vi "API_BINANCE_Execute_Function.vi"(0 "BinanceAPI in":refnum<class "BinanceAPI_.lvclass">, 11 "error in (no error)":errorcluster) -> (4 "BinanceAPI out":refnum<class "BinanceAPI_.lvclass">, 6 "Header":string, 8 "Body":string, 14 "REST API URL":string, 15 "error out":errorcluster)   [LabVIEW 2022 SP3, in "BinanceAPI_.lvclass"]
uses:
  BinanceAPI_.lvclass
  BinanceAPI_.lvclass/BinanceAPI_.ctl
  <vilib>/httpClient/PUTBuffer.vi
  <vilib>/httpClient/POSTBuffer.vi
  <vilib>/University of Leeds/SHA256/SHA256.lvlib
  <vilib>/httpClient/LabVIEWHTTPClient.lvlib
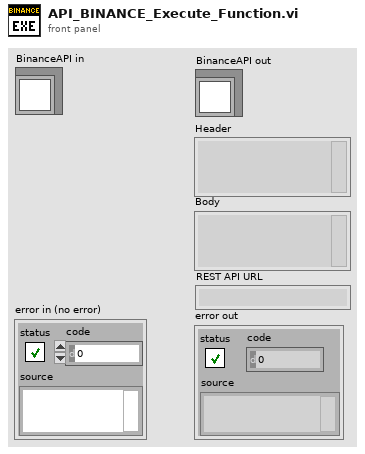
[diagram p1: front panel]
types:
  T1 = enum16{"SPOT", "USDT_FUTURES", "COIN_FUTURES", "VANILLA"}
  T2 = typedef "LabVIEWHTTPClient.lvlib/ClientHandle.ctl" = refnum<k1>
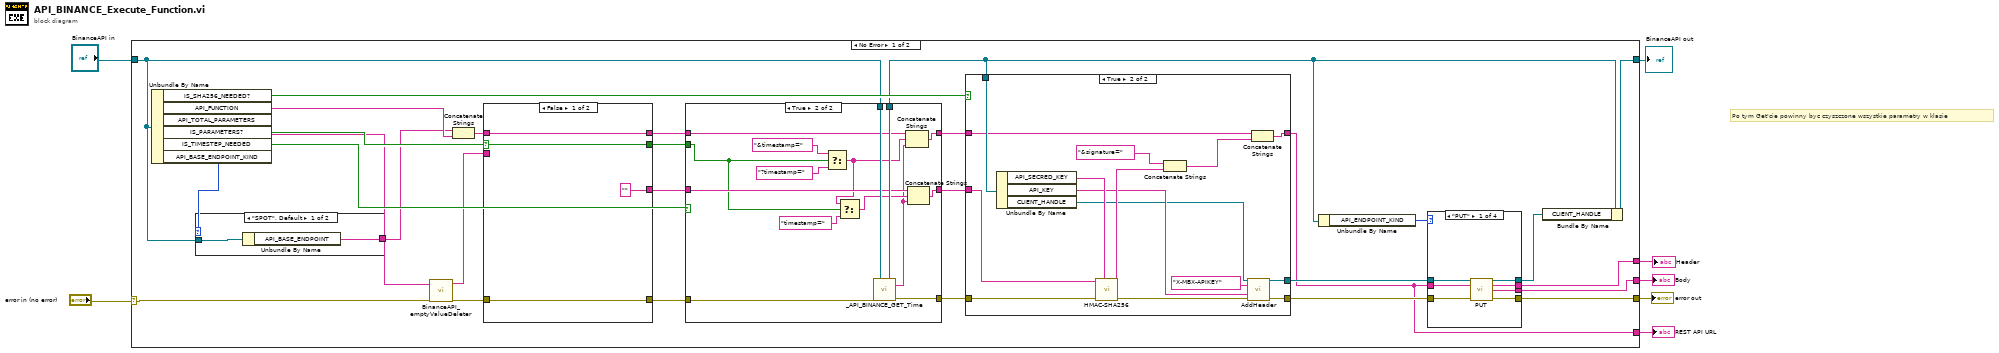
[diagram p0: block diagram]
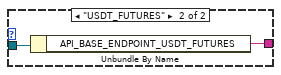
[diagram p2: hidden frame]
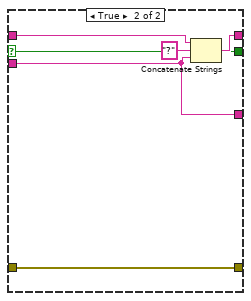
[diagram p4: hidden frame]
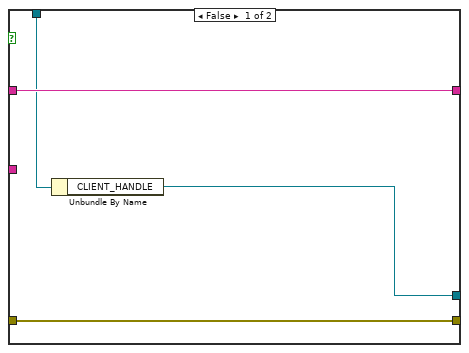
[diagram p5: hidden frame]
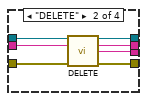
[diagram p6: hidden frame]
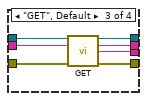
[diagram p7: hidden frame]
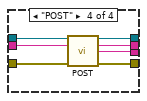
[diagram p8: hidden frame]
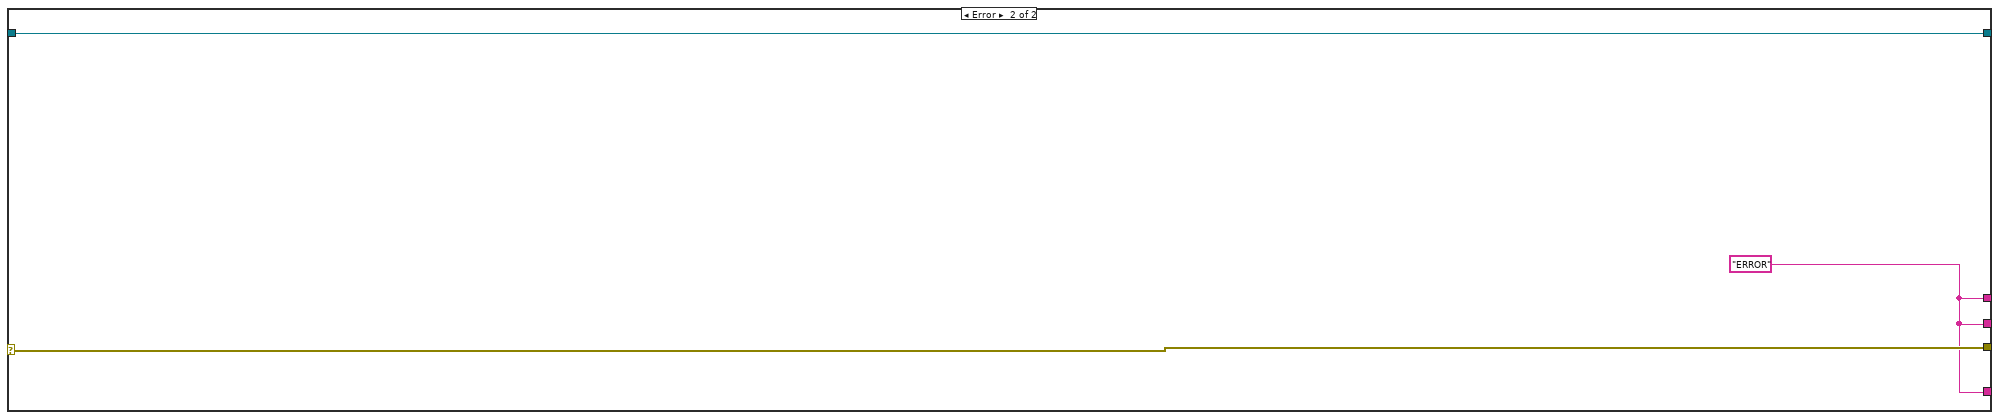
[diagram p9: hidden frame]
diagram:
  # "Po tym Get'cie powinny byc czyszczone wszystkie parametry w klasie"
  n1 = case shown="No Error" "error in (no error)" {
    selector: "error in (no error)" -> [w9 w119]
    tunnel: [w34 w119] -> w6
    tunnel: [w36 w118] -> w1
    tunnel: "BinanceAPI in" -> [w15 w118]
    tunnel: [w18 w117] -> w5
    tunnel: [w17 w117] -> w4
    tunnel: [w12 w117] -> w3
    frame No Error {
      n2 = Unbundle By Name(w15) -> ("IS_SHA256_NEEDED?"=w29:bool, "API_FUNCTION"=w33:string, "API_TOTAL_PARAMETERS"=w11:string, "IS_PARAMETERS?"=w28:bool, "IS_TIMESTEP_NEEDED"=w24:bool, "API_BASE_ENDPOINT_KIND"=w16:T1)
      n3 = case shown="\"SPOT\", Default" w16 {
        tunnel: w15 -> [w38 w40]
        tunnel: [w37 w39] -> w14
        frame "SPOT", Default {
          n4 = Unbundle By Name(w38) -> ("API_BASE_ENDPOINT"=w37:string)
        }
        frame "USDT_FUTURES" {
          n5 = Unbundle By Name(w40) -> ("API_BASE_ENDPOINT_USDT_FUTURES"=w39:string)
        }
      }
      n6 = call "BinanceAPI_emptyValueDeleter.vi"("error in (no error)"=w9, "API_TOTAL_PARAMETERS with NaN"=w11) -> ("error out"=w8:errorcluster, "API_TOTAL_PARAMETERS withOUT NaN"=w10:string)  [unwired: 8 in]
      n7 = Concatenate Strings(w14, w33) -> (w31:string)
      n8 = case shown="False" w28 {
        selector: w28 -> [w60 w64]
        tunnel: w31 -> [w63 w69]
        tunnel: [w63 w67] -> w20
        tunnel: [w62 w66] -> w26
        tunnel: w10 -> [_ w65]
        tunnel: w8 -> [w62 w66]
        tunnel: ["" ("API_TOTAL_PARAMETERS withOUT NaN") w65] -> w23
        tunnel: [w60 w64] -> w13
        frame False {
        }
        frame True {
          n9 = Concatenate Strings(w69, "?" ("string"), w65) -> (w67:string)
        }
      }
      n10 = case shown="True" w24 {
        tunnel: w26 -> [w44 w59]
        tunnel: [w44 w58] -> w25
        tunnel: w23 -> [w42 w55]
        tunnel: w15 -> [w43 w57]
        tunnel: [w43 w56] -> w22
        tunnel: [w42 w54] -> w21
        tunnel: w20 -> [w41 w53]
        tunnel: [w41 w52] -> w19
        tunnel: w13 -> [_ w49]
        frame False {
        }
        frame True {
          n11 = Select(t="&timestamp=" ("string"), s=w49, f="?timestamp=" ("string")) -> (s? t:f=w48:string)
          n12 = Select(t=w48, s=w49, f="timestamp=" ("string")) -> (s? t:f=w47:string)
          n13 = call "_API_BINANCE_GET_Time.vi"("BinanceAPI_.lvclass"=w57, "error in (no error)"=w59) -> ("BinanceAPI_.lvclass 2"=w56:refnum<class "BinanceAPI_.lvclass">, "Time in seckond from 01.01.1970"=w45:string, "error out"=w58:errorcluster)  [unwired: 10 in, 1 out]
          n14 = Concatenate Strings(w53, w48, w45) -> (w52:string)
          n15 = Concatenate Strings(w55, w47, w45) -> (w54:string)
        }
      }
      n16 = case shown="True" w29 {
        tunnel: w22 -> [w71 w85]
        tunnel: w25 -> [w72 w84]
        tunnel: [w72 w77] -> w30
        tunnel: w19 -> [w73 w83]
        tunnel: [w73 w81] -> w12
        tunnel: [w70 w76] -> w32
        tunnel: w21 -> [_ w75]
        frame False {
          n17 = Unbundle By Name(w71) -> ("CLIENT_HANDLE"=w70:T2)
        }
        frame True {
          n18 = Unbundle By Name(w85) -> ("API_SECRED_KEY"=w88:string, "API_KEY"=w79:string, "CLIENT_HANDLE"=w74:T2)
          n19 = call <vilib>:"HMAC-SHA256.vi"("Key"=w88, "error In"=w84, "String to Encode"=w75) -> ("error Out"=w78:errorcluster, "Hash String"=w87:string)  [unwired: 7 in]
          n20 = Concatenate Strings("&signature=" ("username"), w87) -> (w82:string)
          n21 = call <vilib>:"AddHeader.vi"("client handle"=w74, "header"="X-MBX-APIKEY" ("Header_name"), "value"=w79, "error in (no error)"=w78) -> ("client handle out"=w76:T2, "error out"=w77:errorcluster)  [unwired: 10 in]
          n22 = Concatenate Strings(w83, w82) -> (w81:string)
        }
      }
      n23 = Unbundle By Name(w22) -> ("API_ENDPOINT_KIND"=w27:enum16{"POST", "DELETE", "GET", "PUT"})
      n24 = case shown="\"PUT\"" w27 {
        tunnel: [w91 w100 w109 w110] -> w17
        tunnel: [w89 w98 w108 w113] -> w35
        tunnel: [w92 w101 w107 w112] -> w34
        tunnel: w30 -> [w93 w96 w106 w115]
        tunnel: w32 -> [w95 w97 w105 w116]
        tunnel: [w90 w99 w104 w111] -> w18
        tunnel: w12 -> [w94 w102 w103 w114]
        frame "PUT" {
          n25 = call-poly <vilib>:"PUT.vi"("client handle"=w95, "url"=w94, "error in (no error)"=w93) -> ("client handle out"=w89:T2, "headers"=w90:string, "body"=w91:string, "error out"=w92:errorcluster)  [unwired: 9 in]
        }
        frame "DELETE" {
          n26 = call <vilib>:"DELETE.vi"("client handle"=w97, "url"=w102, "error in (no error)"=w96) -> ("client handle out"=w98:T2, "headers"=w99:string, "body"=w100:string, "error out"=w101:errorcluster)  [unwired: 9 in]
        }
        frame "GET", Default {
          n27 = call <vilib>:"GET.vi"("client handle"=w105, "url"=w103, "error in (no error)"=w106) -> ("client handle out"=w108:T2, "headers"=w104:string, "body"=w109:string, "error out"=w107:errorcluster)  [unwired: 9 in]
        }
        frame "POST" {
          n28 = call-poly <vilib>:"POST.vi"("client handle"=w116, "url"=w114, "error in (no error)"=w115) -> ("client handle out"=w113:T2, "headers"=w111:string, "body"=w110:string, "error out"=w112:errorcluster)  [unwired: 9 in]
        }
      }
      n29 = Bundle By Name(cluster=w22, "CLIENT_HANDLE"=w35) -> (w36:refnum<class "BinanceAPI_.lvclass">)
    }
    frame Error {
      w117 = "ERROR" ("headers")
    }
  }
  "error out" <- w6
  "Body" <- w4
  "Header" <- w5
  "REST API URL" <- w3
  "BinanceAPI out" <- w1
